vi "给所有修饰上色.vi"(8 "错误输入（无错误）":errorcluster, 9 "前景色":u32(colorbox), 10 "背景色":u32(colorbox), 11 "引用":refnum<vi>) -> (0 "错误输出":errorcluster, 3 "引用输出":refnum<vi>)   [LabVIEW 8.6, in "窗口操作.lvlib"]
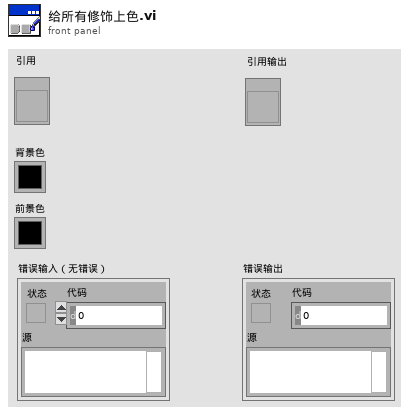
[diagram p1: front panel]
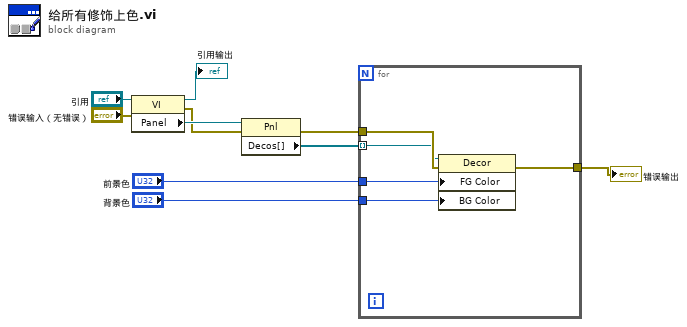
[diagram p0: block diagram]
diagram:
  n1 = property class="VI"(reference="引用", error in="错误输入（无错误）") -> (reference out=→"引用输出":refnum<vi>, error out=w6:errorcluster, "Panel"=w10:refnum<vi>)
  n2 = property class="Pnl"(reference=w10, error in=w6) -> (error out=w4:errorcluster, "Decos[]"=w3:refnum<vi>[])  [unwired: 1 out]
  n3 = for {
    tunnel: "前景色" -> [w15]
    tunnel: "背景色" -> [w14]
    tunnel: [w13] -> w5
    tunnel: w4 -> [w12]
    tunnel: w3 -> [w11] mode=indexing
    n4 = property class="Decor"(reference=w11, error in=w12, "FG Color"=w15, "BG Color"=w14) -> (error out=w13:errorcluster)  [unwired: 1 out]
  }
  "错误输出" <- w5
